vi "ex_CheckMultifileTermCond.vi"(5 "file size (bytes)":i32, 6 "new_file_now":bool, 9 "termination conditions":T1, 11 "Signals":waveform(dbl)[](array[waveform])) -> (3 "start new file?":bool)   [LabVIEW 2017]
uses:
  <vilib>/express/express output/ExFileWriteBlock.llb/ex_NewFileOptions.ctl
  <vilib>/Waveform/WDTOps.llb/WDT Number of Waveform Samples DBL.vi
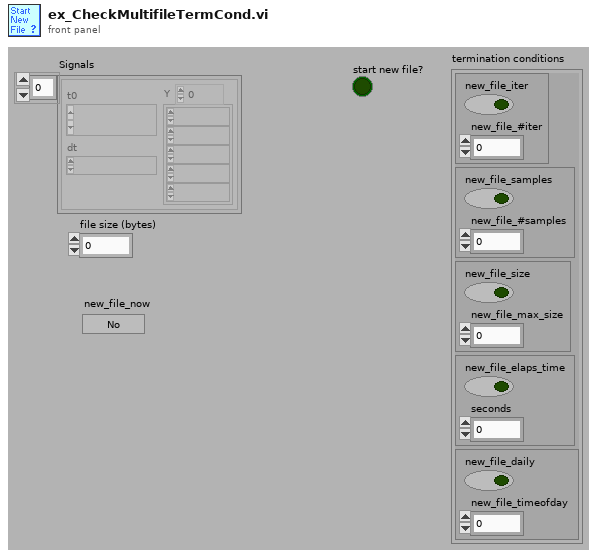
[diagram p1: front panel]
types:
  T1 = typedef "ex_NewFileOptions.ctl" = cluster{cluster{"new_file_iter":bool, "new_file_#iter":i32}, cluster{"new_file_samples":bool, "new_file_#samples":i32}, cluster{"new_file_size":bool, "new_file_max_size":i32}, cluster{"new_file_elaps_time":bool, "seconds":i32}, cluster{"new_file_daily":bool, "new_file_timeofday":i32}}
  T2 = cluster{"new_file_iter":bool, "new_file_#iter":i32}
  T3 = cluster{"new_file_samples":bool, "new_file_#samples":i32}
  T4 = cluster{"new_file_size":bool, "new_file_max_size":i32}
  T5 = cluster{"new_file_elaps_time":bool, "seconds":i32}
  T6 = cluster{"new_file_daily":bool, "new_file_timeofday":i32}
  T7 = cluster{"second":i32, "minute":i32, "hour":i32, "day of month":i32, "month":i32, "year":i32, "day of week":i32, "day of year":i32, "is DST":i32}
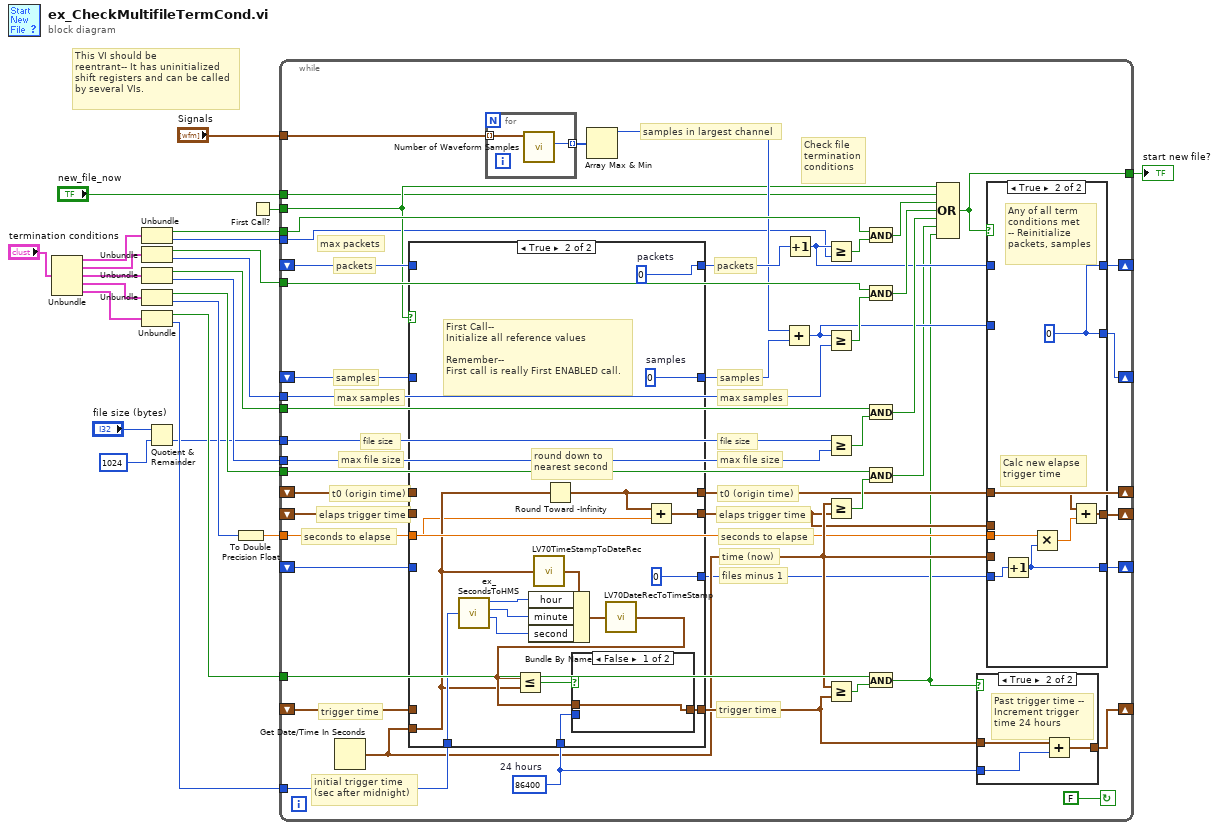
[diagram p0: block diagram]
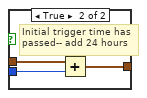
[diagram p5: hidden frame]
diagram:
  # "This VI should be\nreentrant-- It has uninitialized\nshift registers and can be called\nby several VIs."
  n1 = Unbundle("termination conditions") -> (w6:T2, w5:T3, w4:T4, w3:T5, w2:T6)
  n2 = Unbundle(w6) -> ("new_file_iter"=w20:bool, "new_file_#iter"=w23:i32)
  n3 = Unbundle(w5) -> ("new_file_samples"=w11:bool, "new_file_#samples"=w12:i32)
  n4 = Unbundle(w4) -> ("new_file_size"=w18:bool, "new_file_max_size"=w17:i32)
  n5 = Unbundle(w3) -> ("new_file_elaps_time"=w16:bool, "seconds"=w15:i32)
  n6 = Unbundle(w2) -> ("new_file_daily"=w13:bool, "new_file_timeofday"=w19:i32)
  n7 = Quotient & Remainder(x="file size (bytes)", y=1024 ("file size (bytes)")) -> (floor(x/y)=w9:i32)  [unwired: 1 out]
  n8 = To Double Precision Float(number=w15) -> (double precision float=w1:dbl)
  n9 = First Call?() -> (First Call?: T/F=w24:bool)
  n10 = while {
    tunnel: w24 -> [w43]
    tunnel: w23 -> [w39]
    shift-right: [w58] -> _
    shift-left: _ -> [w54]
    tunnel: w12 -> [w72]
    shift-right: [w59] -> _
    shift-left: _ -> [w53]
    tunnel: "new_file_now" -> [w42]
    tunnel: "Signals" -> [w40]
    tunnel: w20 -> [w71]
    tunnel: w11 -> [w56]
    tunnel: w18 -> [w70]
    tunnel: w17 -> [w69]
    tunnel: w16 -> [w68]
    shift-right: [w34] -> _
    shift-left: _ -> [w51]
    shift-right: [w47] -> _
    shift-left: _ -> [w50]
    tunnel: [w30] -> w14
    tunnel: w19 -> [w48]
    tunnel: w13 -> [w67]
    tunnel: w9 -> [w44]
    shift-right: [w33] -> _
    shift-left: _ -> [w35]
    tunnel: w1 -> [w31]
    shift-right: [w26] -> _
    shift-left: _ -> [w25]
    stop <- FALSE continue-if-true
    w45 = u32 86400  # 24 hours
    # "files minus 1"
    # "initial trigger time\n(sec after midnight)"
    # "Check file\ntermination\nconditions"
    # "seconds to elapse"
    # "seconds to elapse"
    # "trigger time"
    # "elaps trigger time"
    # "time (now)"
    # "packets"
    # "samples in largest channel"
    # "t0 (origin time)"
    # "t0 (origin time)"
    # "trigger time"
    # "samples"
    # "file size"
    # "max file size"
    # "max samples"
    # "max packets"
    # "max samples"
    # "elaps trigger time"
    # "max file size"
    # "file size"
    # "samples"
    # "packets"
    n11 = Get Date/Time In Seconds() -> (seconds since 1Jan1904=w36:timestamp)
    n12 = case shown="True" w43 {
      tunnel: [w94 w100] -> w55
      tunnel: w54 -> [w94 _]
      tunnel: w53 -> [w93 _]
      tunnel: [w93 w101] -> w52
      tunnel: w51 -> [w92 _]
      tunnel: [w92 w95] -> w34
      tunnel: w50 -> [w91 _]
      tunnel: w36 -> [_ w98]
      tunnel: w48 -> [_ w111]
      tunnel: [w91 w110] -> w41
      tunnel: w45 -> [_ w109]
      tunnel: w35 -> [w90 _]
      tunnel: [w90 w99] -> w32
      tunnel: w31 -> [_ w97]
      tunnel: [w89 0] -> w27
      tunnel: w25 -> [w89 _]
      frame False {
        # "Not First Call"
      }
      frame True {
        w101 = u32 0  # samples
        w100 = u32 0  # packets
        # "round down to\nnearest second"
        # "First Call--\nInitialize all reference values\n\nRemember--\nFirst call is really First ENABLED call."
        n13 = call <vilib>:"ex_SecondsToHMS.vi"("seconds"=w111) -> ("hours"=w106:i32, "minutes"=w104:i32, "seconds"=w103:i32)  [unwired: 1 out]
        n14 = call <vilib>:"LV70TimeStampToDateRec.vi"("time stamp"=w98) -> ("date time rec"=w107:T7)
        n15 = Bundle By Name(cluster=w107, "hour"=w106, "minute"=w104, "second"=w103) -> (w105:T7)
        n16 = Round Toward -Infinity(1:w98) -> (0:w95:timestamp)
        n17 = call <vilib>:"LV70DateRecToTimeStamp.vi"("date time rec"=w105) -> ("Time Stamp"=w102:timestamp)
        n18 = Less Or Equal?(x=w102, y=w98) -> (x <= y?=w108:bool)
        n19 = case shown="False" w108 {
          tunnel: [w112 w115] -> w110
          tunnel: w109 -> [_ w114]
          tunnel: w102 -> [w112 w113]
          frame False {
          }
          frame True {
            # "Initial trigger time has\npassed-- add 24 hours"
            n20 = Add(x=w113, y=w114) -> (x+y=w115:timestamp)
          }
        }
        n21 = Add(x=w95, y=w97) -> (x+y=w99:timestamp)
      }
    }
    n22 = for {
      tunnel: w40 -> [w116] mode=indexing
      tunnel: [w117] -> w60 mode=indexing
      n23 = call-poly <vilib>:"Number of Waveform Samples.vi"("waveform in"=w116) -> ("number of samples"=w117:i32)  [unwired: 1 in, 9 out]
    }
    n24 = Array Max & Min(array=w60) -> (max value=w49:i32)  [unwired: 3 out]
    n25 = Add(x=w49, y=w52) -> (x+y=w38:u32)
    n26 = Increment(x=w55) -> (x+1=w57:u32)
    n27 = Greater Or Equal?(x=w57, y=w39) -> (x >= y?=w66:bool)
    n28 = Greater Or Equal?(x=w38, y=w72) -> (x >= y?=w64:bool)
    n29 = Greater Or Equal?(x=w44, y=w69) -> (x >= y?=w62:bool)
    n30 = Greater Or Equal?(x=w36, y=w32) -> (x >= y?=w37:bool)
    n31 = Greater Or Equal?(x=w36, y=w41) -> (x >= y?=w46:bool)
    n32 = And(x=w71, y=w66) -> (x .and. y?=w65:bool)
    n33 = And(x=w56, y=w64) -> (x .and. y?=w63:bool)
    n34 = And(x=w70, y=w62) -> (x .and. y?=w61:bool)
    n35 = And(x=w68, y=w37) -> (x .and. y?=w28:bool)
    n36 = And(x=w67, y=w46) -> (x .and. y?=w29:bool)
    n37 = Compound Arithmetic op=OR(w43, w42, w65, w63, w61, w28, w29) -> (w30:bool)
    n38 = case shown="True" w29 {
      tunnel: [w74 w75] -> w47
      tunnel: w45 -> [_ w77]
      tunnel: w41 -> [w74 w76]
      frame False {
      }
      frame True {
        # "Past trigger time --\nIncrement trigger \ntime 24 hours"
        n39 = Add(x=w76, y=w77) -> (x+y=w75:timestamp)
      }
    }
    n40 = case shown="True" w30 {
      tunnel: [w80 w88] -> w59
      tunnel: [w81 w88] -> w58
      tunnel: w57 -> [w81 _]
      tunnel: w38 -> [w80 _]
      tunnel: [w79 w87] -> w33
      tunnel: w32 -> [w79 _]
      tunnel: w31 -> [_ w85]
      tunnel: w36 -> [_ _]
      tunnel: w27 -> [w78 w82]
      tunnel: [w78 w86] -> w26
      tunnel: w34 -> [_ w83]
      frame False {
      }
      frame True {
        w88 = u32 0
        # "Calc new elapse\ntrigger time"
        # "Any of all term \nconditions met\n-- Reinitialize \npackets, samples"
        n41 = Increment(x=w82) -> (x+1=w86:i32)
        n42 = Multiply(x=w85, y=w86) -> (x*y=w84:dbl)
        n43 = Add(x=w83, y=w84) -> (x+y=w87:timestamp)
      }
    }
  }
  "start new file?" <- w14
